vi "Motion_2D_continuous_Scan_Control_signal_Generator_simple_win7.vi"() -> ()   [LabVIEW 2015]
uses:
  Agilent 33XXX Series/Agilent 33XXX Series.lvlib
panel:
  out "Secondary Steps Left":dbl
  out "Current Repetition":dbl
  in  "Number of Repetitions":i32=1 min=1 max=100 step=1
  in  "Burst Pulse Repetition Frequency (Hz)":dbl
  in  "Peak-Peak Amplitude  in Volts":dbl
  in  "Fundamental Frequency in MHz":dbl
  in  "Number of Cycles":i32=1
  in  "VISA resource name":refnum<visa-resource-name>
  out "Elapsed time":dbl
  in  "Primary Motor\nNumber":i32=1 min=1 max=3 step=1
  in  "Secondary Motor\nNumber":i32=1 min=1 max=3 step=1
  in  "Motor Speed (mm/sec)":dbl=10.0 caption="Range:0.1-30 by 0.1" min=0.1 max=30.0 step=0.1
  in  "Raster Scan Length \nPrimary (mm)":dbl
  in  "Step Size \nSecondary  (um)":dbl
  in  "Raster Scan Length \nSecondary  (mm)":dbl
  in  "Operation":string(combo)
  in  "Single Axis Movement":dbl caption="(mm)"
  in  "Motor Number":i32=1 min=1 max=3 step=1
  # "Primary Scan Length MUST be >0\nSecondary Scan Length Must be > or = 0"
  # "+2"
  # "+3"
  # "+1 +1"
  # "MOTION CONTROL"
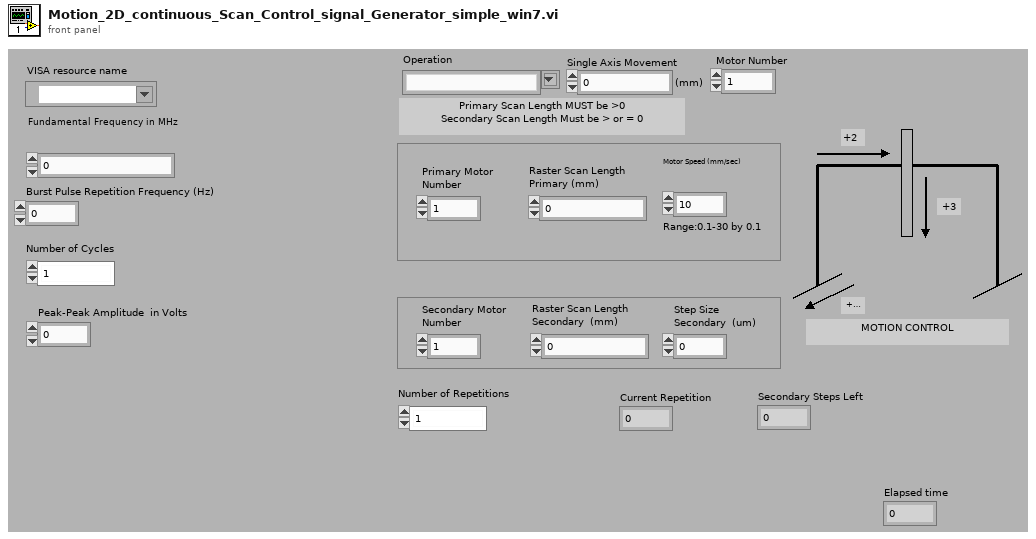
[diagram p1: front panel]
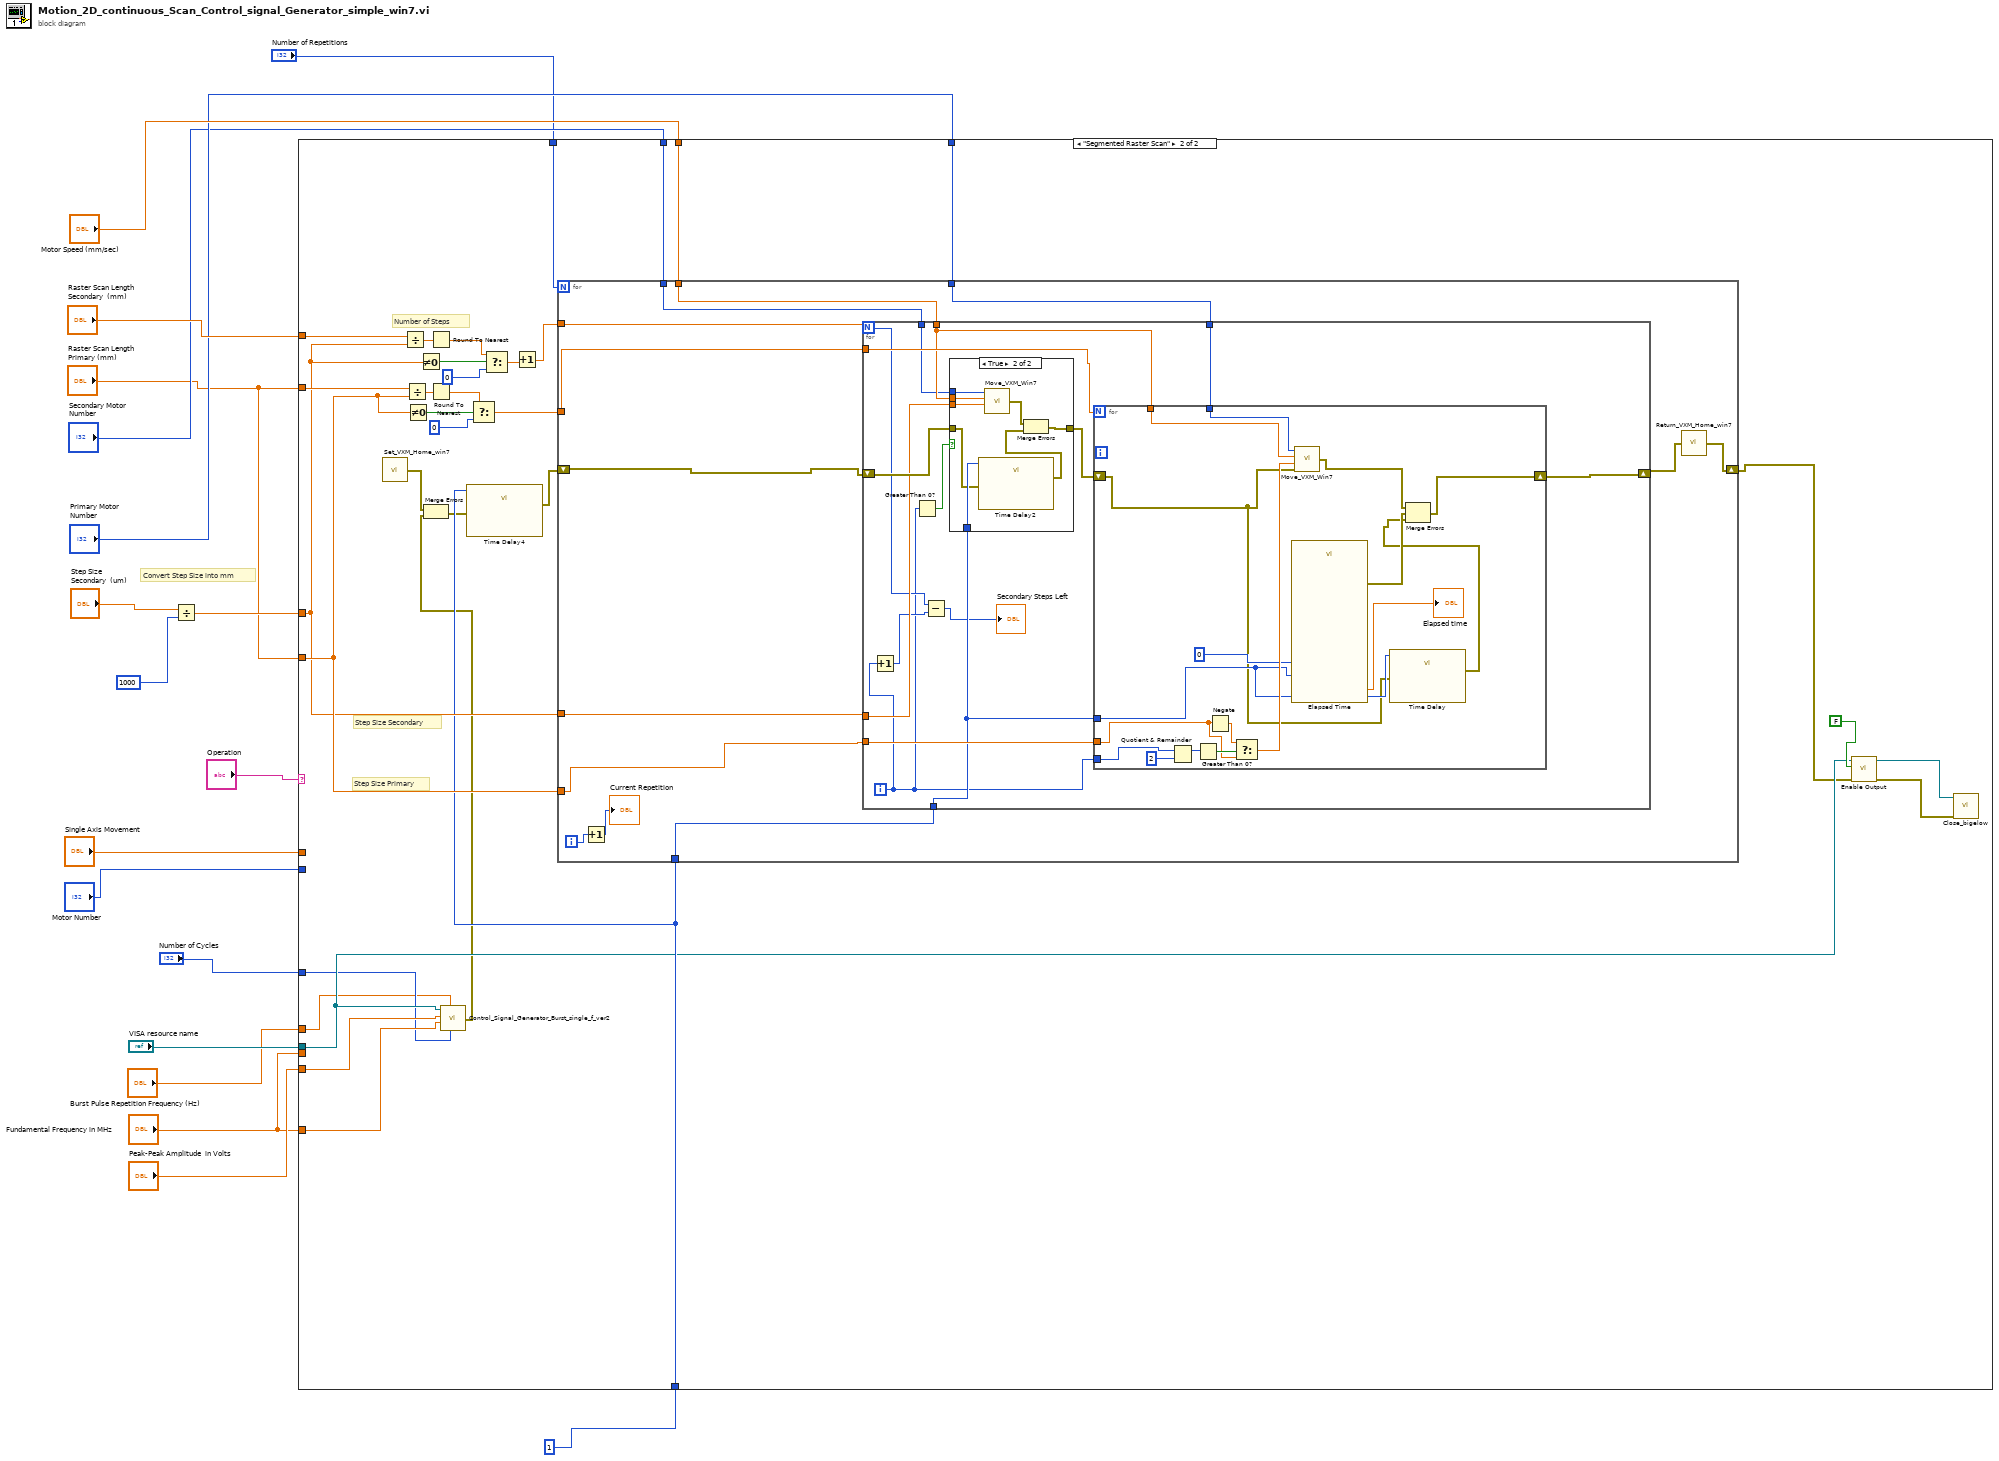
[diagram p0: block diagram]
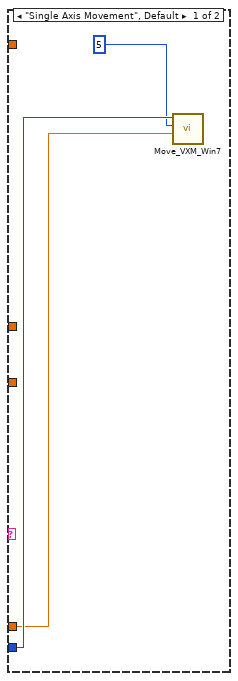
[diagram p2: hidden frame]
diagram:
  # "Convert Step Size into mm"
  n1 = Divide(x="Step Size \nSecondary  (um)", y=1000) -> (x/y=w12:dbl)
  n2 = case shown="\"Segmented Raster Scan\"" "Operation" {
    tunnel: "Raster Scan Length \nSecondary  (mm)" -> [_ w52]
    tunnel: "Raster Scan Length \nPrimary (mm)" -> [_ w51]
    tunnel: w12 -> [_ w37]
    tunnel: "Raster Scan Length \nPrimary (mm)" -> [_ w50]
    tunnel: "Motor Speed (mm/sec)" -> [_ w54]
    tunnel: "Primary Motor\nNumber" -> [_ w53]
    tunnel: "Motor Number" -> [w21 _]
    tunnel: "Single Axis Movement" -> [w20 _]
    tunnel: "Secondary Motor\nNumber" -> [_ w49]
    tunnel: 1 -> [_ w35]
    tunnel: "VISA resource name" -> [_ w29]
    tunnel: "Fundamental Frequency in MHz" -> [_ _]
    tunnel: "Burst Pulse Repetition Frequency (Hz)" -> [_ w24]
    tunnel: "Number of Cycles" -> [_ w26]
    tunnel: "Peak-Peak Amplitude  in Volts" -> [_ w28]
    tunnel: "Fundamental Frequency in MHz" -> [_ w27]
    tunnel: "Number of Repetitions" -> [_ w22]
    frame "Single Axis Movement", Default {
      n3 = call "Move_VXM_Win7.vi"("Single Axis Movement (mm)"=w20, "Motor Speed (mm/sec)"=5, "Motor Number"=w21) -> ()  [unwired: 1 in, 1 out]
    }
    frame "Segmented Raster Scan" {
      # "Step Size Primary"
      # "Step Size Secondary"
      # "Number of Steps"
      n4 = call "Set_VXM_Home_win7.vi"() -> ("error out"=w33:errorcluster)  [unwired: 1 in]
      n5 = Divide(x=w52, y=w37) -> (x/y=w47:dbl)
      n6 = Divide(x=w51, y=w50) -> (x/y=w48:dbl)
      n7 = Not Equal To 0?(x=w50) -> (x != 0?=w46:bool)
      n8 = Not Equal To 0?(x=w37) -> (x != 0?=w43:bool)
      n9 = Round To Nearest(number=w47) -> (nearest integer value=w41:dbl)
      n10 = Round To Nearest(number=w48) -> (nearest integer value=w45:dbl)
      n11 = call "Control_Signal_Generator_Burst_single_f_ver2.vi"("Number of Cycles"=w26, "Burst Pulse Repetition Frequency (Hz)"=w24, "Fundamental Frequency in MHz"=w27, "Voltage Peak-Peak (V)"=w28, "VISA resource name"=w29) -> ("error out"=w25:errorcluster)  [unwired: 1 in]
      n12 = Merge Errors(w33, w25) -> (w34:errorcluster)
      n13 = call "Time Delay4"("error in (no error)"=w34, "Delay Time (s)"=w35) -> ("error out"=w36:errorcluster)  [unwired: 9 in]
      n14 = Select(t=w45, s=w46, f=0) -> (s? t:f=w39:dbl)
      n15 = Select(t=w41, s=w43, f=0) -> (s? t:f=w40:dbl)
      n16 = Increment(x=w40) -> (x+1=w38:dbl)
      n17 = for {
        N: w22 -> [_]
        tunnel: w54 -> [w63]
        tunnel: w53 -> [w67]
        tunnel: w50 -> [w59]
        tunnel: w49 -> [w66]
        tunnel: w39 -> [w65]
        tunnel: w38 -> [w64]
        tunnel: w35 -> [w62]
        tunnel: w37 -> [w60]
        shift-right: [w57] -> w23
        shift-left: w36 -> [w61]
        i -> [w56]
        n18 = Increment(x=w56) -> (x+1=→"Current Repetition":i32)
        n19 = for {
          N: w64 -> [w71]
          tunnel: w63 -> [w76]
          shift-right: [w73] -> w58
          shift-left: w61 -> [w78]
          tunnel: w60 -> [w77]
          tunnel: w65 -> [w82]
          tunnel: w67 -> [w81]
          tunnel: w59 -> [w80]
          tunnel: w66 -> [w75]
          tunnel: w62 -> [w74]
          i -> [w68]
          n20 = Increment(x=w68) -> (x+1=w70:i32)
          n21 = Greater Than 0?(x=w68) -> (x > 0?=w79:bool)
          n22 = Subtract(x=w71, y=w70) -> (x-y=→"Secondary Steps Left":i32)
          n23 = case shown="True" w79 {
            tunnel: [w83 w84] -> w72
            tunnel: w78 -> [w83 w87]
            tunnel: w77 -> [_ w91]
            tunnel: w76 -> [_ w90]
            tunnel: w75 -> [_ w89]
            tunnel: w74 -> [_ w88]
            frame False {
            }
            frame True {
              n24 = call "Time Delay2"("error in (no error)"=w87, "Delay Time (s)"=w88) -> ("error out"=w85:errorcluster)  [unwired: 9 in]
              n25 = call "Move_VXM_Win7.vi"("Single Axis Movement (mm)"=w91, "Motor Speed (mm/sec)"=w90, "Motor Number"=w89) -> ("error out"=w86:errorcluster)  [unwired: 1 in]
              n26 = Merge Errors(w86, w85) -> (w84:errorcluster)
            }
          }
          n27 = for {
            N: w82 -> [_]
            tunnel: w76 -> [w103]
            tunnel: w81 -> [w102]
            tunnel: w80 -> [w104]
            tunnel: w68 -> [w100]
            tunnel: w74 -> [w94]
            shift-right: [w95] -> w73
            shift-left: w72 -> [w93]
            n28 = Quotient & Remainder(x=w100, y=2) -> (x-y*floor(x/y)=w107:i32)  [unwired: 1 out]
            n29 = Greater Than 0?(x=w107) -> (x > 0?=w106:bool)
            n30 = Negate(x=w104) -> (-x=w105:dbl)
            n31 = Select(t=w105, s=w106, f=w104) -> (s? t:f=w101:dbl)
            n32 = call "Elapsed Time"("Time Target (s)"=w94, "Set Start Time (s)"=0) -> ("Elapsed Time (s)"=→"Elapsed time":dbl, "error out"=w96:errorcluster)  [unwired: 10 in, 6 out]
            n33 = call "Move_VXM_Win7.vi"("error in (no error)"=w93, "Single Axis Movement (mm)"=w101, "Motor Speed (mm/sec)"=w103, "Motor Number"=w102) -> ("error out"=w97:errorcluster)
            n34 = call "Time Delay"("error in (no error)"=w93, "Delay Time (s)"=w94) -> ("error out"=w92:errorcluster)  [unwired: 9 in]
            n35 = Merge Errors(w97, w96, w92) -> (w95:errorcluster)
          }
        }
        n36 = call "Return_VXM_Home_win7.vi"("error in (no error)"=w58) -> ("error out"=w57:errorcluster)
      }
      n37 = call "Enable Output.vi"("error in (no error)"=w23, "Enable Output  (T: Enable)"=FALSE, "VISA resource name"=w29) -> ("error out"=w31:errorcluster, "VISA resource name out"=w32:refnum<visa-resource-name>)  [unwired: 7 in]
      n38 = call "Close_bigelow.vi"("error in (no error)"=w31, "VISA resource name"=w32) -> ()  [unwired: 9 in, 1 out]
    }
  }
